vi "Test Create a Logger with TDMS Sink.vi"(11 "Test Case In":refnum<class "TDMS Sink.lvclass">) -> (0 "error out":errorcluster, 3 "Test Case Out":refnum<class "TDMS Sink.lvclass">)   [LabVIEW 2020, in "TDMS Sink.lvclass"]
uses:
  TDMS Sink.lvclass
  C:/Program Files (x86)/National Instruments/LabVIEW 2020/vi.lib/Astemes/LUnit/Test Case.lvclass
  Source/Type Defs/Debug Level.ctl
  <vilib>/Astemes/LUnit/Test Case.lvclass/Test Case.ctl
  c87a3b73-c721-4c84-b9a9-a8ecc75a75ee.vi
  3e02e809-91ce-4d23-a366-20949767ee2e.vi
  961363e7-8f67-43de-bc46-14219c673455.vi
  <vilib>/Astemes/LUnit/Core/LUnit Test Case/Private/Append Fail Result.vi
  <vilib>/Astemes/LUnit/Core/LUnit Test Case/Private/Append Pass Result.vi
  c87a3b73-c721-4c84-b9a9-a8ecc75a75ee.vi/9c5d11cd-9439-4240-a1ee-d9baace9c924.vi
  3e02e809-91ce-4d23-a366-20949767ee2e.vi/9c5d11cd-9439-4240-a1ee-d9baace9c924.vi
  961363e7-8f67-43de-bc46-14219c673455.vi/9c5d11cd-9439-4240-a1ee-d9baace9c924.vi
  <vilib>/Astemes/LUnit/Core/LUnit Test Case/Private/Run In UI.vi
  <vilib>/Utility/error.llb/Clear Errors.vi
  Source/Sinks/TDMS Sink/TDMS Sink.lvclass
  C:/Users/hughe_cx/Documents/05_repos/LVLog/Source/Sinks/Sink/Sink.lvclass
  TDMS Sink.lvclass/TDMS Sink.ctl
  Source/LV Log.lvlib
  Source/Logger/Logger.lvclass
  <vilib>/Astemes/LUnit/Test Case.lvclass
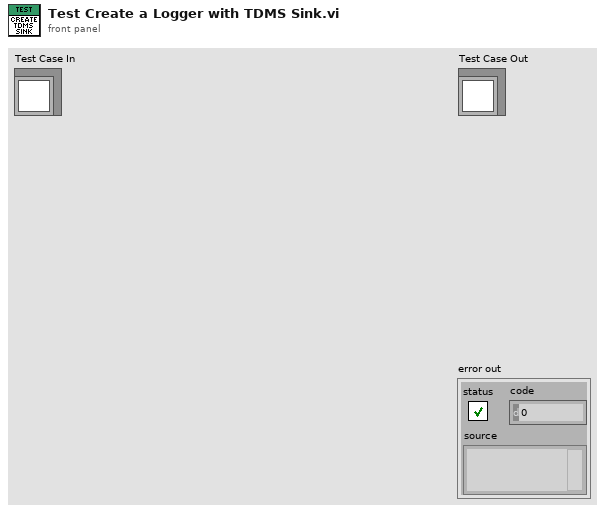
[diagram p1: front panel]
types:
  T1 = typedef "LV Log.lvlib/Debug Level.ctl" = enum16{"DEFAULT", "DEBUG", "INFO", "WARN", "ERROR", "FATAL"}
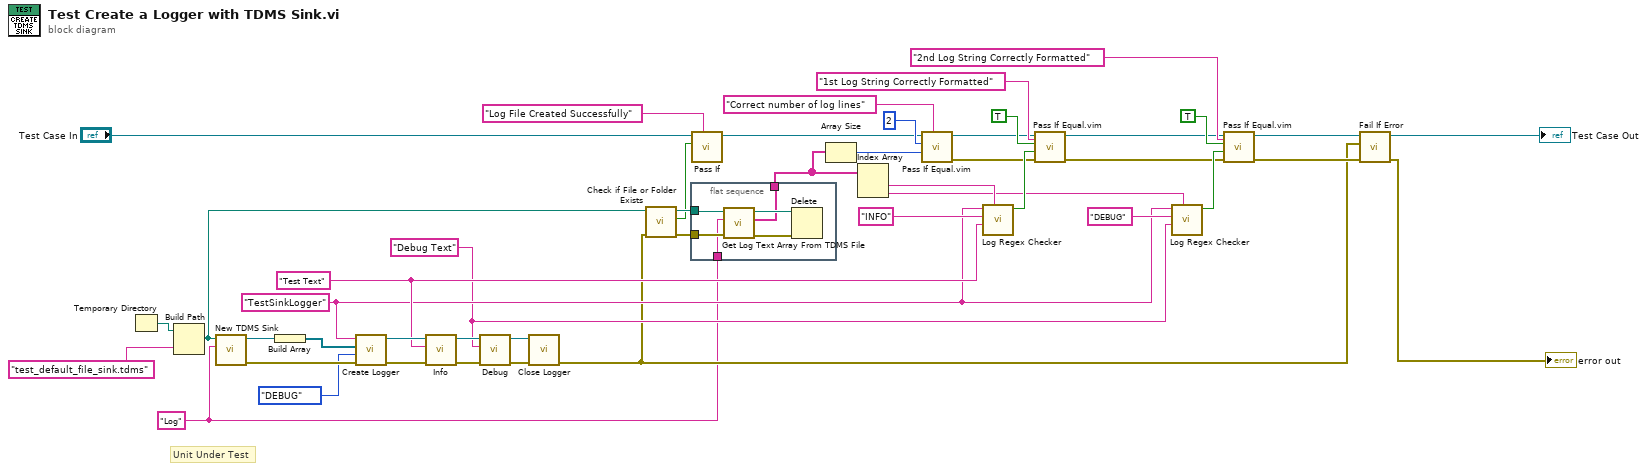
[diagram p0: block diagram]
diagram:
  w7 = "Log" ("Group Name")
  w31 = "Debug Text" ("Log Text")
  w41 = "Test Text" ("Log Text")
  w32 = "TestSinkLogger" ("Name")
  # "Unit Under Test"
  n1 = Temporary Directory() -> (w46:path)
  n2 = Build Path(base path=w46, name or relative path="test_default_file_sink.tdms" ("format string")) -> (appended path=w8:path)
  n3 = call "New TDMS Sink.vi"("Group Name"=w7, "TDMS File Path"=w8) -> ("error out"=w10:errorcluster, "TDMS out"=w9:refnum<class "TDMS Sink.lvclass">)  [unwired: 8 in]
  n4 = Build Array(w9) -> (w6:refnum<class "TDMS Sink.lvclass">[])
  n5 = call "Create Logger.vi"("error in (no error)"=w10, "Debug Level (Default)"=Debug_Level."DEBUG", "Sinks (Default)"=w6, "Name"=w32) -> ("error out"=w45:errorcluster, "Logger out"=w44:refnum<class "Logger.lvclass">)  [unwired: 6 in]
  n6 = call "Info.vi"("error in (no error)"=w45, "Log Text"=w41, "Logger in"=w44) -> ("error out"=w40:errorcluster, "Logger out"=w39:refnum<class "Logger.lvclass">)  [unwired: 6 in, 1 out]
  n7 = call "Debug.vi"("error in (no error)"=w40, "Log Text"=w31, "Logger in"=w39) -> ("error out"=w13:errorcluster, "Logger out"=w12:refnum<class "Logger.lvclass">)  [unwired: 6 in, 1 out]
  n8 = call "Close Logger.vi"("error in (no error)"=w13, "Logger in"=w12) -> ("error out"=w11:errorcluster)  [unwired: 9 in]
  n9 = call <vilib>:"Check if File or Folder Exists.vi"("error in (no error)"=w11, "path"=w8) -> ("error out"=w17:errorcluster, "file or folder exists?"=w15:bool, "dup path"=w18:path)  [unwired: 7 in]
  n10 = flat-sequence {
    tunnel: w18 -> [w51]
    tunnel: [w48] -> w25
    tunnel: w17 -> [w52]
    tunnel: w7 -> [w47]
    frame #0 {
      n11 = call "Get Log Text Array From TDMS File.vi"("error in"=w52, "Group Name"=w47, "Log File Path in"=w51) -> ("error out"=w49:errorcluster, "Log Text Array"=w48:string[], "Log File Path out"=w50:path)  [unwired: 6 in]
      n12 = Delete(path (use dialog)=w50, error in=w49) -> ()  [unwired: 3 in, 3 out]
    }
  }
  n13 = call <vilib>:"Pass If.vi"("Description"="Log File Created Successfully", "Pass?"=w15, "LUnit Test Case In"="Test Case In") -> ("LUnit Test Case Out"=w16:refnum<class "TDMS Sink.lvclass">)  [unwired: 7 in, 1 out]
  n14 = Array Size(array=w25) -> (size(s)=w24:i32)
  n15 = Index Array(array=w25) -> (element #1=w30:string, element #2=w29:string)  [unwired: 2 in]
  n16 = call "Pass If Equal.vim"("Description"="Correct number of log lines", "Actual"=w24, "Expected"=2, "LUnit Test Case In"=w16) -> ("error out"=w19:errorcluster, "LUnit Test Case Out"=w26:refnum<class "TDMS Sink.lvclass">)  [unwired: 6 in]
  n17 = call "Log Regex Checker.vi"("Log String"=w30, "Expected Log Text (Any)"=w41, "Expected Log Level (Any)"="INFO", "Expected Logger Name (Any)"=w32) -> ("Math Found"=w37:bool)  [unwired: 5 in, 2 out]
  n18 = call "Pass If Equal.vim"("Description"="1st Log String Correctly Formatted", "error in (no error)"=w19, "Actual"=w37, "Expected"=TRUE, "LUnit Test Case In"=w26) -> ("error out"=w20:errorcluster, "LUnit Test Case Out"=w28:refnum<class "TDMS Sink.lvclass">)  [unwired: 5 in]
  n19 = call "Log Regex Checker.vi"("Log String"=w29, "Expected Log Text (Any)"=w31, "Expected Log Level (Any)"="DEBUG", "Expected Logger Name (Any)"=w32) -> ("Math Found"=w36:bool)  [unwired: 5 in, 2 out]
  n20 = call "Pass If Equal.vim"("Description"="2nd Log String Correctly Formatted", "error in (no error)"=w20, "Actual"=w36, "Expected"=TRUE, "LUnit Test Case In"=w28) -> ("error out"=w21:errorcluster, "LUnit Test Case Out"=w27:refnum<class "TDMS Sink.lvclass">)  [unwired: 5 in]
  n21 = call <vilib>:"Fail If Error.vi"("error in (no error)"=w21, "Assert error"=w11, "LUnit Test Case In"=w27) -> ("error out"=→"error out":errorcluster, "LUnit Test Case Out"=→"Test Case Out":refnum<class "TDMS Sink.lvclass">)  [unwired: 7 in]
